vi "counter test2.vi"() -> ()   [LabVIEW 2015]
panel:
  out "output cluster":cluster{"data":dbl, "data":u8}
  in  "Stop Button":bool
  out "Enum":T1(ring)
  out "Boolean array":bool[](array[boolean])
  out "exit":bool=TRUE
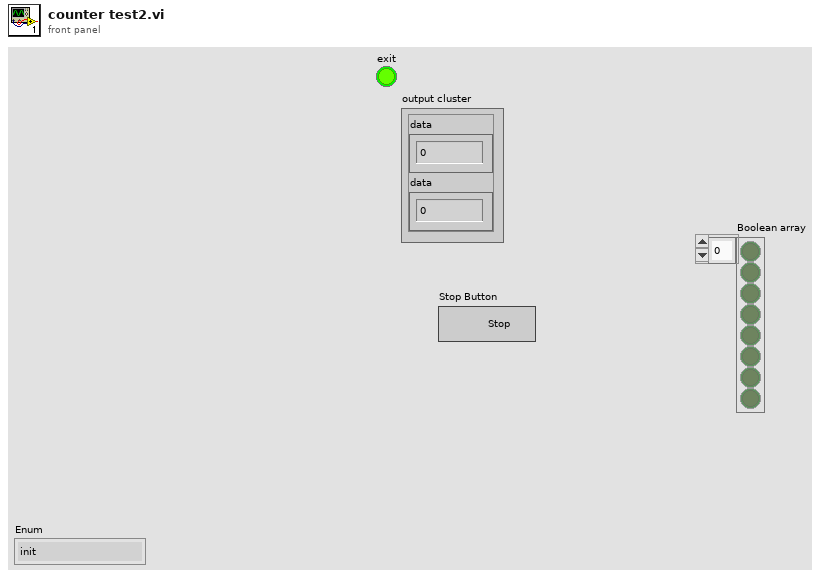
[diagram p1: front panel]
types:
  T1 = enum16{"init", "wait", "start", "do", "stop", "exit"}
  T2 = enum16{"init", "config", "start", "read", "stop"}
  T3 = enum16{"init", "config", "start", "write", "stop"}
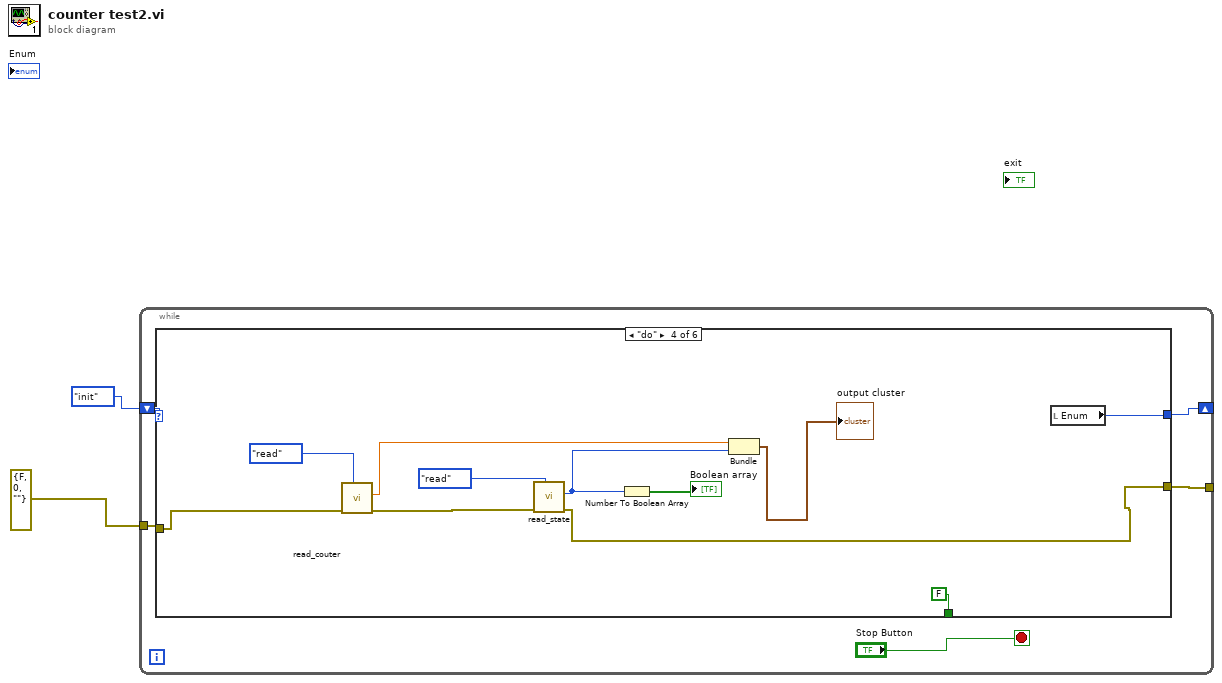
[diagram p0: block diagram]
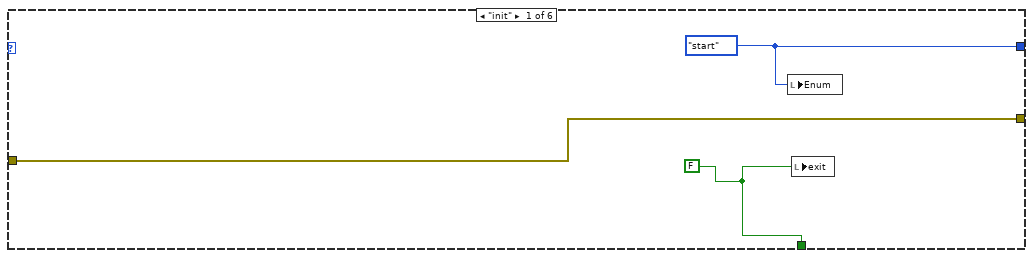
[diagram p2: hidden frame]
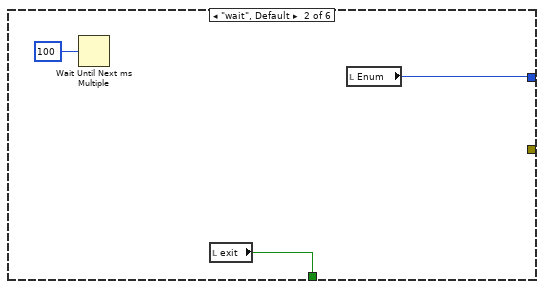
[diagram p3: hidden frame]
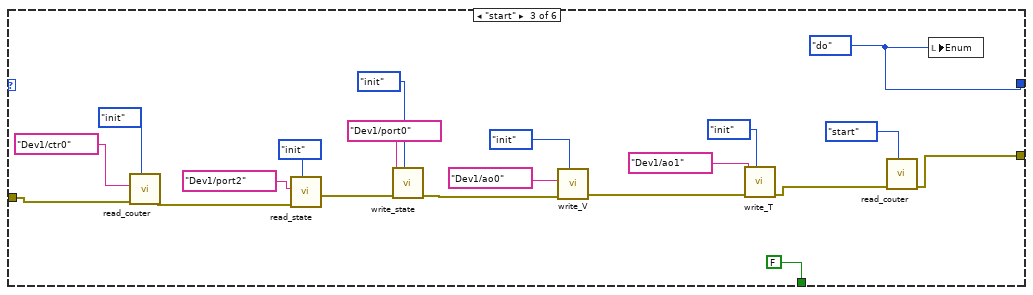
[diagram p4: hidden frame]
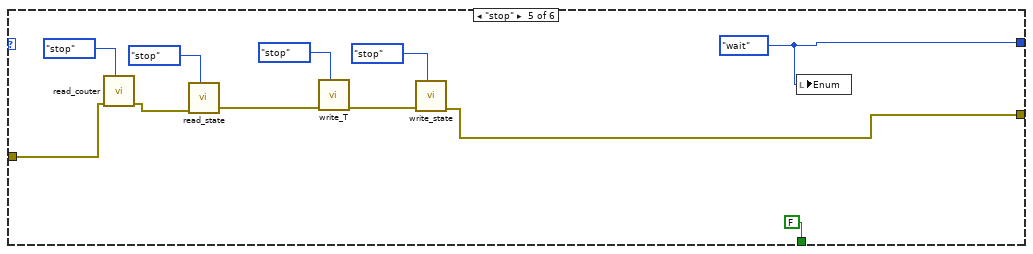
[diagram p5: hidden frame]
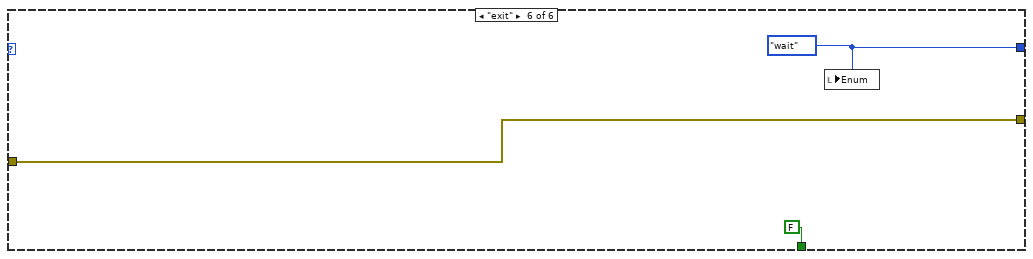
[diagram p6: hidden frame]
diagram:
  n1 = while {
    shift-right: [w6] -> _
    shift-left: T1."init" ("Enum") -> [w7]
    tunnel: errorcluster {"status"=FALSE, "code"=0, "source"=""} ("error out") -> [w5]
    tunnel: [w4] -> _
    stop <- "Stop Button" stop-if-true
    n2 = case shown="\"do\"" w7 {
      tunnel: [w10 w13 FALSE ("exit") FALSE ("exit") FALSE ("exit") FALSE ("exit")] -> _
      tunnel: [w9 w12 w32 w43 w54 w57] -> w6
      tunnel: w5 -> [w8 _ w28 w42 w53 w56]
      tunnel: [w8 _ w19 w34 w49 w56] -> w4
      frame "init" {
        w9 = T1."start" ("Enum")
        w10 = FALSE
        n3 = local write "Enum"(w9) -> ()
        n4 = local write "exit"(w10) -> ()
      }
      frame "wait", Default {
        n5 = Wait Until Next ms Multiple(millisecond multiple=u32 100) -> ()  [unwired: 1 out]
        n6 = local read "exit"() -> (w13:bool)
        n7 = local read "Enum"() -> (w12:T1)
      }
      frame "start" {
        w32 = T1."do" ("Enum")
        n8 = call "read_couter.vi"("Enum"=T2."init", "error in"=w28, "counter"=tag "Dev1/ctr0") -> ("error out"=w21:errorcluster)  [unwired: 7 in, 1 out]
        n9 = call "read_state.vi"("Enum"=T2."init", "error in"=w21, "lines"=tag "Dev1/port2") -> ("error out"=w27:errorcluster)  [unwired: 7 in, 1 out]
        n10 = call "write_state.vi"("Enum"=T3."init", "error in"=w27, "lines"=tag "Dev1/port0") -> ("error out"=w25:errorcluster)  [unwired: 7 in]
        n11 = call "write_V.vi"("Enum"=T3."init", "error in"=w25, "physical channels"=tag "Dev1/ao0") -> ("error out"=w24:errorcluster)  [unwired: 8 in]
        n12 = call "write_T.vi"("Enum"=T3."init", "error in"=w24, "physical channels"=tag "Dev1/ao1") -> ("error out"=w20:errorcluster)  [unwired: 8 in]
        n13 = call "read_couter.vi"("Enum"=T2."start", "error in"=w20) -> ("error out"=w19:errorcluster)  [unwired: 8 in, 1 out]
        n14 = local write "Enum"(w32) -> ()
      }
      frame "do" {
        n15 = call "read_couter.vi"("Enum"=T2."read", "error in"=w42) -> ("error out"=w41:errorcluster, "data"=w38:dbl)  [unwired: 8 in]
        n16 = call "read_state.vi"("Enum"=T2."read", "error in"=w41) -> ("error out"=w34:errorcluster, "data"=w36:u8)  [unwired: 8 in]
        n17 = Number To Boolean Array(number=w36) -> (Boolean array=→"Boolean array":bool[])
        n18 = Bundle("data"=w38, "data"=w36) -> (→"output cluster":cluster{"data":dbl, "data":u8})  [unwired: 1 in]
        n19 = local read "Enum"() -> (w43:T1)
      }
      frame "stop" {
        w54 = T1."wait" ("Enum")
        n20 = call "read_couter.vi"("Enum"=T2."stop", "error in"=w53) -> ("error out"=w52:errorcluster)  [unwired: 8 in, 1 out]
        n21 = call "read_state.vi"("Enum"=T2."stop", "error in"=w52) -> ("error out"=w51:errorcluster)  [unwired: 8 in, 1 out]
        n22 = call "write_T.vi"("Enum"=T3."stop", "error in"=w51) -> ("error out"=w50:errorcluster)  [unwired: 9 in]
        n23 = call "write_state.vi"("Enum"=T3."stop", "error in"=w50) -> ("error out"=w49:errorcluster)  [unwired: 8 in]
        n24 = local write "Enum"(w54) -> ()
      }
      frame "exit" {
        w57 = T1."wait" ("Enum")
        n25 = local write "Enum"(w57) -> ()
      }
    }
  }
